vi "PAQmem_ReadData.vi"(6 "TagsIndices":i32[](array[numeric]), 8 "error in (no error)":errorcluster, 9 "Time-End":timestamp, 10 "Time-Start":timestamp, 11 "PAQ-memory in":refnum<class "PAQ-memory.lvclass">) -> (0 "error out":errorcluster, 2 "PAQ_section":T1, 3 "PAQ-memory out":refnum<class "PAQ-memory.lvclass">)   [LabVIEW 2020, in "Sgraph_lib_V1.lvlib" / "PAQ-memory.lvclass"]
doc: "Read some data from a PAQ memory Layer"
uses:
  PAQ-memory.lvclass
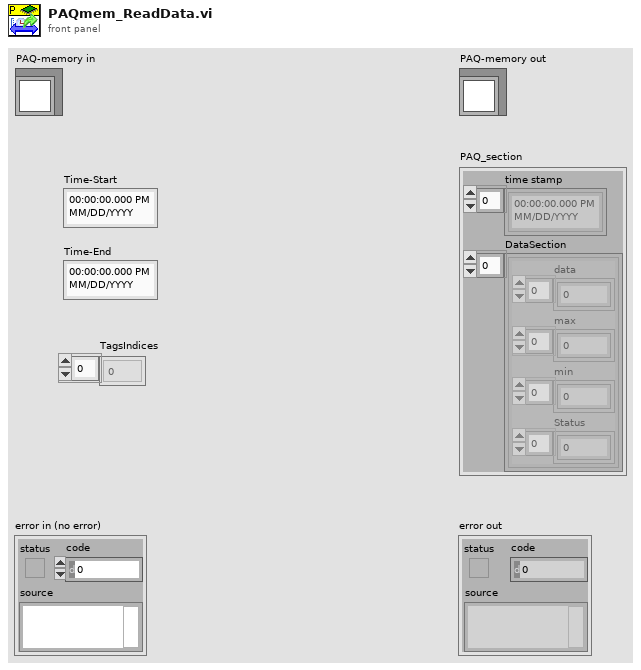
[diagram p1: front panel]
types:
  T1 = cluster{"time stamp":timestamp[], "DataSection":cluster{"data":dbl[], "max":dbl[], "min":dbl[], "Status":u32[]}[]}
  T2 = cluster{"data":dbl[], "max":dbl[], "min":dbl[], "Status":u32[]}[]
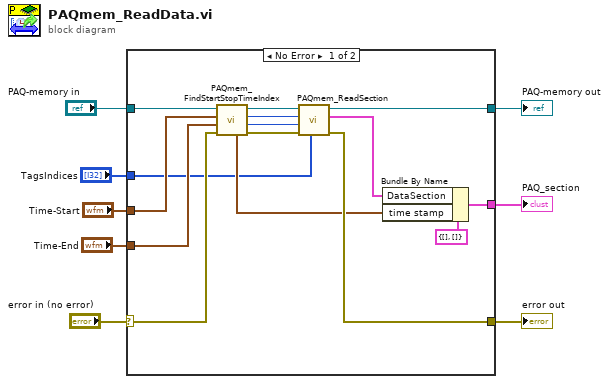
[diagram p0: block diagram]
diagram:
  n1 = case shown="No Error" "error in (no error)" {
    selector: "error in (no error)" -> [w20 w25]
    tunnel: [w17 w25] -> w7
    tunnel: [w14 w24] -> w5
    tunnel: "PAQ-memory in" -> [w23 w24]
    tunnel: "Time-Start" -> [w22 _]
    tunnel: "Time-End" -> [w21 _]
    tunnel: "TagsIndices" -> [w10 _]
    tunnel: [w9 _] -> w1
    frame No Error {
      n2 = call "PAQmem_FindStartStopTimeIndex.vi"("error in (no error)"=w20, "End-time"=w21, "Start-time"=w22, "PAQ-memory in"=w23) -> ("error out"=w18:errorcluster, "Size"=w15:i32, "Start"=w16:i32, "PAQ-memory out"=w19:refnum<class "PAQ-memory.lvclass">, "time"=w11:timestamp[])  [unwired: 3 in]
      n3 = call "PAQmem_ReadSection.vi"("TagsIndices"=w10, "error in (no error)"=w18, "Length"=w15, "Start"=w16, "PAQ-memory in"=w19) -> ("error out"=w17:errorcluster, "DataSection"=w12:T2, "PAQ-memory out"=w14:refnum<class "PAQ-memory.lvclass">)  [unwired: 4 in]
      n4 = Bundle By Name(cluster=T1 {"time stamp"=[], "DataSection"=[]} ("PAQ_section"), "DataSection"=w12, "time stamp"=w11) -> (w9:T1)
    }
    frame Error {
    }
  }
  "error out" <- w7
  "PAQ-memory out" <- w5
  "PAQ_section" <- w1
